vi "LJUD_eTCValues.vi"(5 "aResetCounters":i32[](array[numeric]), 6 "aTimerValuesWrite":dbl[](array[numeric]) format="%.2f", 7 "aReadCounters":i32[](array[numeric]), 8 "error in":errorcluster, 9 "aUpdateResetTimers":i32[](array[numeric]), 10 "aReadTimers":i32[](array[numeric]), 11 "Handle In":i32) -> (0 "error out":errorcluster, 1 "aCounterValues":dbl[](array[numeric]) format="%.2f", 2 "aTimerValuesRead":dbl[](array[numeric]) format="%.2f", 3 "Handle Out":i32)   [LabVIEW 2021]
doc: "This is an e-function that can update\nand read all the timers and counters\nin a single call. A somewhat complex\nfunction, but can help reinforce the\ninteraction between the different timers\nand counters on the device.\n\nSee Sections 4.2 and 4.3 of the device's\ndatasheet for more information."
uses:
  labjackud.dll
panel:
  # "This is an e-function that can update\nand read all the timers and counters\nin a single call.  A somewhat complex\nfunction, but can help reinforce the\ninteraction between the different timers\nand counters on the device.\n\nSee Sections 4.2 and 4.3 of the device's\ndatasheet for more information."
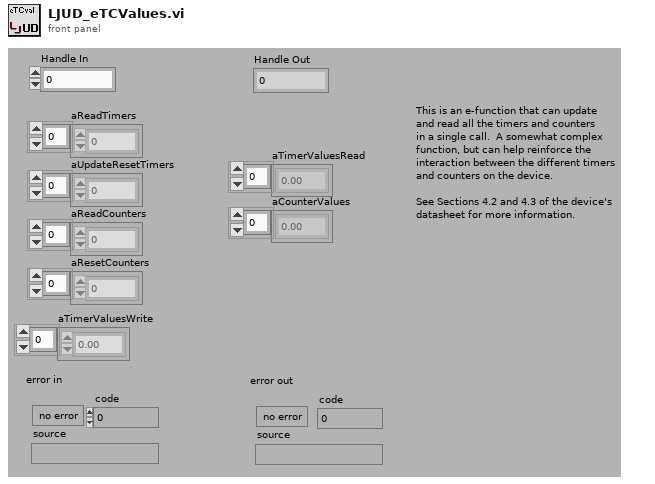
[diagram p1: front panel]
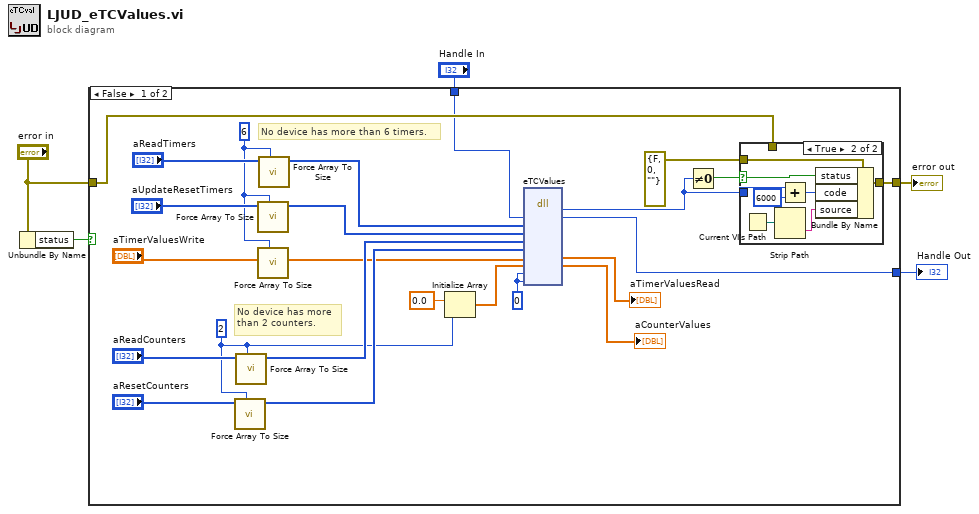
[diagram p0: block diagram]
diagram:
  n1 = Unbundle By Name("error in") -> ("status"=w4:bool)
  n2 = case shown="False" w4 {
    tunnel: [w26 w40] -> w5
    tunnel: "error in" -> [w25 w40]
    tunnel: "Handle In" -> [w10 w39]
    tunnel: [w9 w39] -> w1
    frame False {
      w6 = 6 ("# Elements")
      w15 = 2 ("# Elements")
      w22 = 0 ("GoError")
      # "No device has more\nthan 2 counters."
      # "No device has more than 6 timers."
      n3 = call "Force Array To Size.vi"("# Elements"=w15, "I32 Array In"="aResetCounters") -> ("I32 Array Out"=w18:i32[])  [unwired: 6 in, 3 out]
      n4 = call "Force Array To Size.vi"("# Elements"=w15, "I32 Array In"="aReadCounters") -> ("I32 Array Out"=w19:i32[])  [unwired: 6 in, 3 out]
      n5 = call "Force Array To Size.vi"("# Elements"=w6, "I32 Array In"="aUpdateResetTimers") -> ("I32 Array Out"=w11:i32[])  [unwired: 6 in, 3 out]
      n6 = call "Force Array To Size.vi"("# Elements"=w6, "DBL Array In"="aTimerValuesWrite") -> ("DBL Array Out"=w7:dbl[])  [unwired: 6 in, 3 out]
      n7 = call "Force Array To Size.vi"("# Elements"=w6, "I32 Array In"="aReadTimers") -> ("I32 Array Out"=w12:i32[])  [unwired: 6 in, 3 out]
      n8 = Initialize Array(0.0 ("Element Data"), w15) -> (w14:dbl[])
      n9 = dll-call lib="labjackud.dll" fn="eTCValues"("Handle"=w10, "aReadTimers"=w12, "aUpdateResetTimers"=w11, "aReadCounters"=w19, "aResetCounters"=w18, "aTimerValues"=w7, "aCounterValues"=w14, "Reserved1"=w22, "Reserved2"=w22) -> (w27:i32, "Handle"=w9:i32, "aTimerValues"=→"aTimerValuesRead":dbl[], "aCounterValues"=→"aCounterValues":dbl[])  [unwired: 9 in, 2 out]
      n10 = Not Equal To 0?(x=w27) -> (x != 0?=w28:bool)
      n11 = case shown="True" w28 {
        selector: w28 -> [_ w37]
        tunnel: [w30 w38] -> w26
        tunnel: errorcluster {"status"=FALSE, "code"=0, "source"=""} ("error IO") -> [_ w36]
        tunnel: w27 -> [_ w32]
        tunnel: w25 -> [w30 _]
        frame False {
        }
        frame True {
          n12 = Current VI's Path() -> (path=w34:path)
          n13 = Strip Path(path=w34) -> (name=w35:string)  [unwired: 1 out]
          n14 = Add(x=w32, y=6000) -> (x+y=w33:i32)
          n15 = Bundle By Name(cluster=w36, "status"=w37, "code"=w33, "source"=w35) -> (w38:errorcluster)
        }
      }
    }
    frame True {
    }
  }
  "error out" <- w5
  "Handle Out" <- w1
